vi "File_Module.vi"(7 "Command":T3, 8 "error in (no error)":errorcluster, 9 "datosEnsayo":T2={"TIEMPO_MIN"=1.0, "S1_TEMPERATURA_C"=1.0, "S2_TEMPERATURA_C"=1.0, "S3_TEMPERATURA_C"=0.0, "S4_TEMPERATURA_C"=0.0, "S5_TEMPERATURA_C"=0.0, "ROT_SETPOINT_RPM"=0.0, "ROT_VELOCIDAD_RPM"=0.0, "ROT_PAR_NM"=0.0, "ROT_TEMPERATURA_C"=0.0} {"ROT_TEMPERATURA_C" format="%.2f"; "S5_TEMPERATURA_C" format="%.2f"; "S4_TEMPERATURA_C" format="%.2f"; "S3_TEMPERATURA_C" format="%.2f"; "ROT_PAR_NM" format="%.2f"; "ROT_VELOCIDAD_RPM" format="%.2f"; "ROT_SETPOINT_RPM" format="%.2f"; "S2_TEMPERATURA_C" format="%.2f"; "S1_TEMPERATURA_C" format="%.2f"; "TIEMPO_MIN" format="%.2f"}, 11 "Window":T1={"Nombre ensayo"="Nombre", "Muestra"="Fluido", "Promedios"=0, "Frecuencia adq(s)"=0.0, "Tiempo medida(min) "=0.0} {"Frecuencia adq(s)" format="%.3f"}) -> (0 "error out":errorcluster, 2 "selected path":path)   [LabVIEW 2017]
uses:
  File_Module Control.ctl
  CRISTALIZADOR_datosEnsayo.ctl
  CRISTALIZADOR_parametrosMedida.ctl
panel:
  out "Cabeceras":string[](array[string])
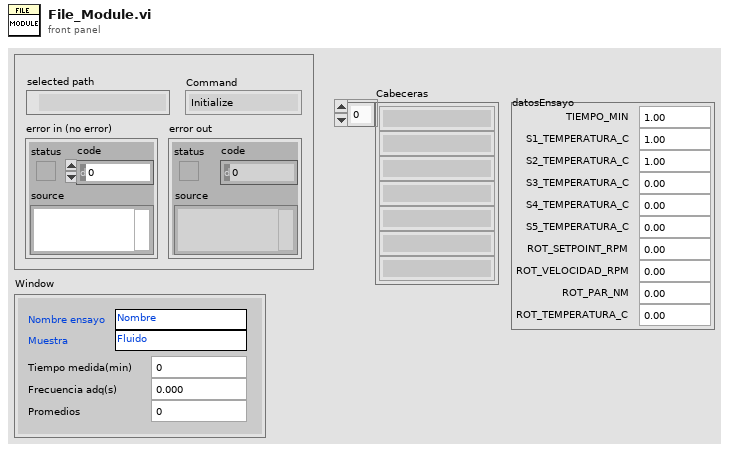
[diagram p1: front panel]
types:
  T1 = typedef "CRISTALIZADOR_parametrosMedida.ctl" = cluster{"Nombre ensayo":string, "Muestra":string, "Promedios":u16, "Frecuencia adq(s)":dbl, "Tiempo medida(min) ":dbl}
  T2 = typedef "CRISTALIZADOR_datosEnsayo.ctl" = cluster{"TIEMPO_MIN":dbl, "S1_TEMPERATURA_C":dbl, "S2_TEMPERATURA_C":dbl, "S3_TEMPERATURA_C":dbl, "S4_TEMPERATURA_C":dbl, "S5_TEMPERATURA_C":dbl, "ROT_SETPOINT_RPM":dbl, "ROT_VELOCIDAD_RPM":dbl, "ROT_PAR_NM":dbl, "ROT_TEMPERATURA_C":dbl}
  T3 = typedef "File_Module Control.ctl" = enum16{"Initialize", "Save Head", "Save Data", "Shutdown"}
  T4 = enum16{"open", "replace", "create", "open or create", "replace or create", "replace or create with confirmation"}
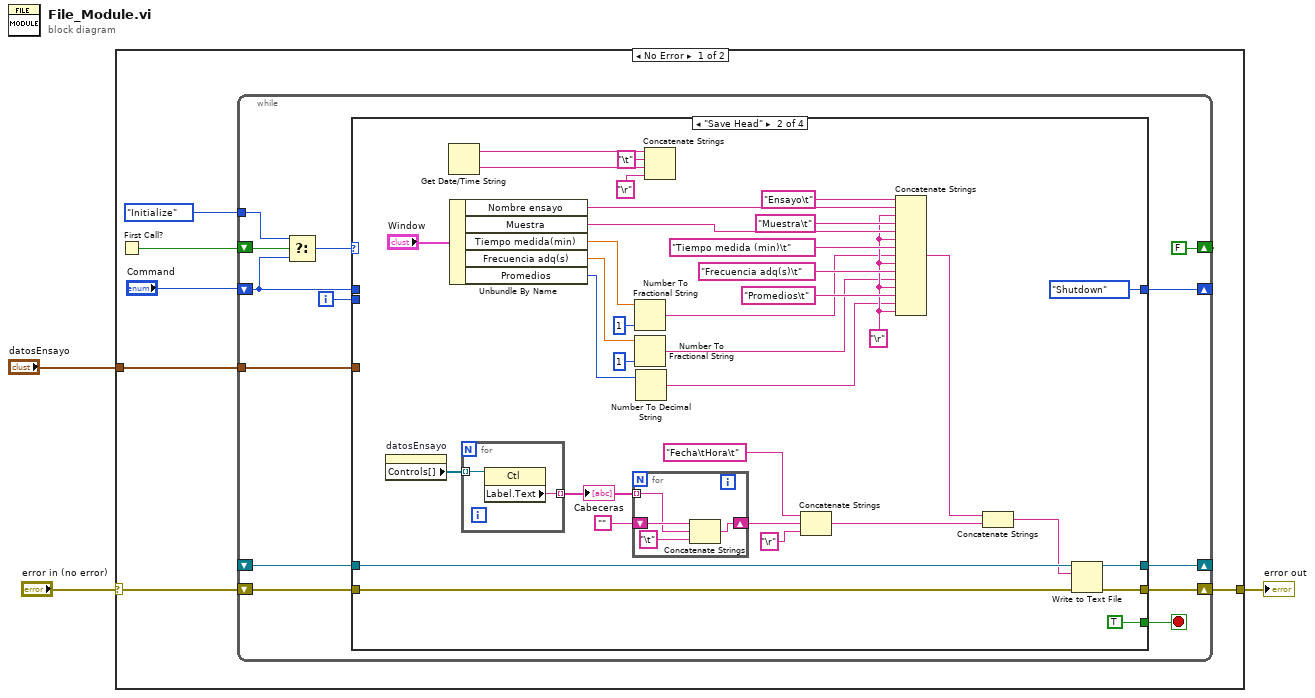
[diagram p0: block diagram]
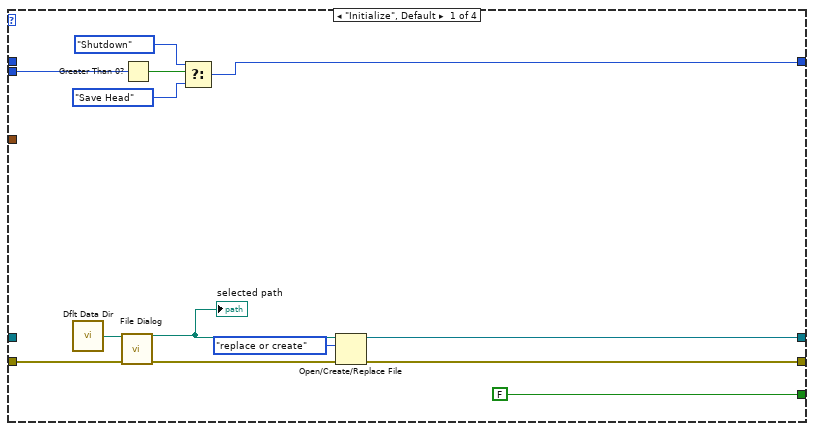
[diagram p2: hidden frame]
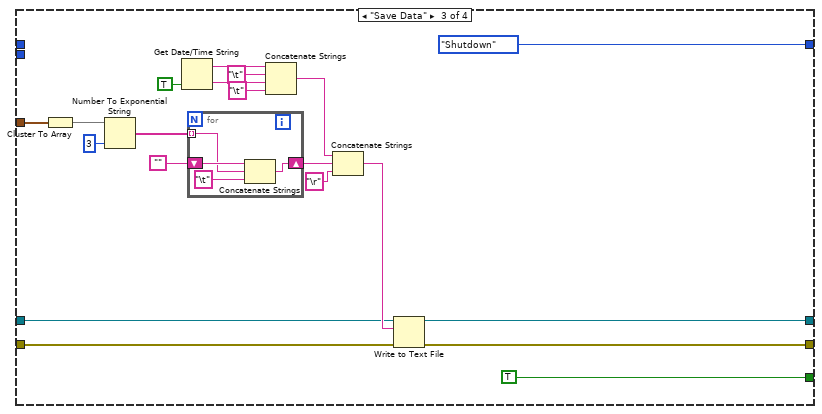
[diagram p3: hidden frame]
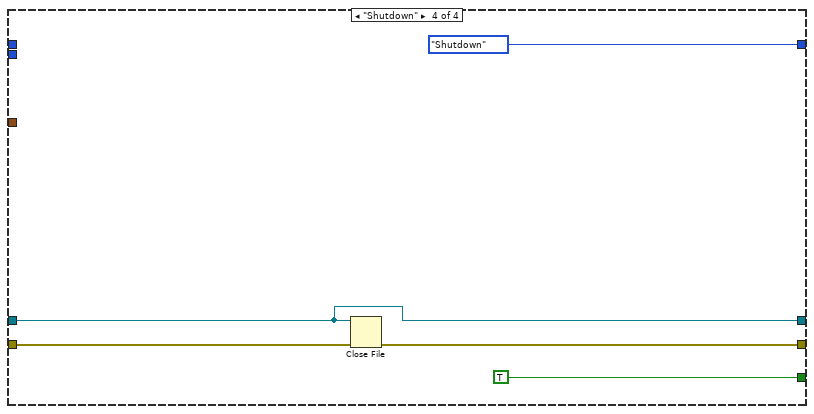
[diagram p4: hidden frame]
diagram:
  n1 = case shown="No Error" "error in (no error)" {
    selector: "error in (no error)" -> [w7 w107]
    tunnel: [w6 w107] -> w2
    tunnel: "datosEnsayo" -> [w4 _]
    frame No Error {
      n2 = First Call?() -> (First Call?: T/F=w9:bool)
      n3 = while {
        shift-right: [w14] -> _
        shift-left: "Command" -> [w15]
        shift-right: [w17] -> w6
        shift-left: w7 -> [w18]
        shift-right: [FALSE ("First Call?: T/F")] -> _
        shift-left: w9 -> [w22]
        tunnel: File_Module_Control."Initialize" ("t") -> [w21]
        shift-right: [w11] -> _
        shift-left: _ -> [w12]
        tunnel: w4 -> [w10]
        i -> [w13]
        stop <- w19 stop-if-true
        n4 = Select(t=w21, s=w22, f=w15) -> (s? t:f=w20:T3)
        n5 = case shown="\"Save Head\"" w20 {
          tunnel: [FALSE TRUE TRUE TRUE] -> w19
          tunnel: w18 -> [w28 w67 w88 w104]
          tunnel: [w24 w66 w87 w103] -> w17
          tunnel: w15 -> [_ _ _ _]
          tunnel: [w34 File_Module_Control."Shutdown" ("t") File_Module_Control."Shutdown" File_Module_Control."Shutdown"] -> w14
          tunnel: w13 -> [w32 _ _ _]
          tunnel: w12 -> [_ w69 w84 w102]
          tunnel: [w23 w68 w86 w102] -> w11
          tunnel: w10 -> [_ _ w90 _]
          frame "Initialize", Default {
            n6 = call <vilib>:"Dflt Data Dir.vi"() -> ("App:Default Data Directory"=w29:path)
            n7 = call "File Dialog"("start path"=w29, "error in"=w28) -> ("selected path"=w26:path, "error out"=w25:errorcluster)  [unwired: 10 in, 2 out]
            "selected path" <- w26
            n8 = Greater Than 0?(x=w32) -> (x > 0?=w31:bool)
            n9 = Select(t=File_Module_Control."Shutdown", s=w31, f=File_Module_Control."Save Head" ("t")) -> (s? t:f=w34:T3)
            n10 = Open/Create/Replace File(file path (use dialog)=w26, error in=w25, operation (0:open)=T4."replace or create") -> (refnum out=w23:refnum<file>, error out=w24:errorcluster)  [unwired: 3 in, 1 out]
          }
          frame "Save Head" {
            w49 = "\r" ("string")
            n11 = property on="datosEnsayo" class="Clust (strict)"() -> ("Controls[]"=w65:refnum<vi>[])  [unwired: 2 in, 2 out]
            n12 = Get Date/Time String() -> (date string=w38:string, time string=w37:string)  [unwired: 3 in]
            n13 = Unbundle By Name("Window") -> ("Nombre ensayo"=w55:string, "Muestra"=w53:string, "Tiempo medida(min)"=w45:dbl, "Frecuencia adq(s)"=w44:dbl, "Promedios"=w43:u16)
            n14 = for {
              tunnel: w65 -> [w77] mode=indexing
              tunnel: [w76] -> w60 mode=indexing
              n15 = property class="Ctl"(reference=w77) -> ("Label.Text"=w76:string)  [unwired: 1 in, 2 out]
            }
            "Cabeceras" <- w60
            n16 = for {
              tunnel: w60 -> [w74] mode=indexing
              shift-right: [w73] -> w64
              shift-left: "" -> [w75]
              n17 = Concatenate Strings(w75, w74, "\t" ("string")) -> (w73:string)
            }
            n18 = Number To Fractional String(number=w45, precision (6)=i16 1) -> (F-format string=w40:string)  [unwired: 2 in]
            n19 = Number To Fractional String(number=w44, precision (6)=i16 1) -> (F-format string=w41:string)  [unwired: 2 in]
            n20 = Number To Decimal String(number=w43) -> (decimal integer string=w42:string)  [unwired: 1 in]
            n21 = Concatenate Strings(w38, "\t" ("string"), w37, "\r" ("string")) -> ()  [unwired: 1 out]
            n22 = Concatenate Strings("Fecha\tHora\t" ("string"), w64, "\r" ("string")) -> (w47:string)
            n23 = Concatenate Strings("Ensayo\t" ("string"), w55, w49, "Muestra\t" ("string"), w53, w49, "Tiempo medida (min)\t" ("string"), w40, w49, "Frecuencia adq(s)\t" ("string"), w41, w49, "Promedios\t" ("string"), w42, w49) -> (w48:string)
            n24 = Concatenate Strings(w48, w47) -> (w46:string)
            n25 = Write to Text File(file (use dialog)=w69, text=w46, error in=w67) -> (refnum out=w68:refnum<file>, error out=w66:errorcluster)  [unwired: 1 in, 1 out]
          }
          frame "Save Data" {
            n26 = Cluster To Array(cluster=w90) -> (array=w91:dbl[])
            n27 = Number To Exponential String(number=w91, precision (6)=i16 3) -> (E-format string=w89:string[])  [unwired: 2 in]
            n28 = Get Date/Time String(want seconds? (F)=TRUE) -> (date string=w80:string, time string=w79:string)  [unwired: 2 in]
            n29 = for {
              tunnel: w89 -> [w100] mode=indexing
              shift-right: [w99] -> w95
              shift-left: "" -> [w101]
              n30 = Concatenate Strings(w101, w100, "\t" ("string")) -> (w99:string)
            }
            n31 = Concatenate Strings(w80, "\t" ("string"), w79, "\t" ("string")) -> (w83:string)
            n32 = Concatenate Strings(w83, w95, "\r" ("string")) -> (w85:string)
            n33 = Write to Text File(file (use dialog)=w84, text=w85, error in=w88) -> (refnum out=w86:refnum<file>, error out=w87:errorcluster)  [unwired: 1 in, 1 out]
          }
          frame "Shutdown" {
            n34 = Close File(refnum=w102, error in=w104) -> (error out=w103:errorcluster)  [unwired: 1 out]
          }
        }
      }
    }
    frame Error {
    }
  }
  "error out" <- w2
